vi "Ultrasonic Sensor simulationfirebase.(GroupDinithi).vi"() -> ()   [LabVIEW 2022 SP3]
uses:
  <vilib>/Analysis/2dsp.llb/Integral Method.ctl
  <vilib>/DAQmx/read.llb/DAQmx Read (Analog Wfm 1Chan NSamp).vi
  <vilib>/DAQmx/write.llb/DAQmx Write (Digital Bool 1Line 1Point).vi
  <vilib>/DAQmx/create/channels.llb/DAQmx Create Channel (DO-Digital Output).vi
  <vilib>/DAQmx/miscellaneous.llb/DAQmx Fill In Error Info.vi
  <vilib>/DAQmx/create/channels.llb/DAQmx Create Channel (AI-Voltage-Basic).vi
  <vilib>/DAQmx/configure/timing.llb/DAQmx Timing (Sample Clock).vi
  <vilib>/httpClient/PUTBuffer.vi
  <vilib>/Analysis/NI_AALPro.lvlib
  <vilib>/httpClient/LabVIEWHTTPClient.lvlib
panel:
  out "Numeric":dbl
  out "body":string
  in  "Cluster":T1
  out "Waveform Graph":waveform(dbl)(graph)
  in  "Number of Samples":dbl
  in  "sampling frequency":dbl
  in  "DAQmx Physical Channel 2":tag
  in  "DAQmx Physical Channel":tag
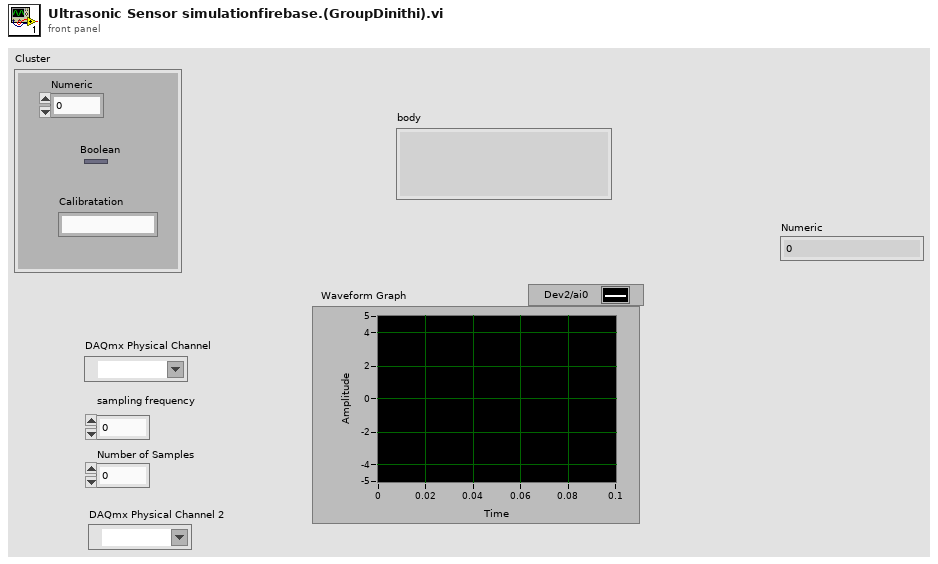
[diagram p1: front panel]
types:
  T1 = cluster{"Numeric":dbl, "Calibratation":string, "Boolean":bool}
  T2 = typedef "NI_AALPro.lvlib/Integral Method.ctl" = i32
  T3 = typedef "LabVIEWHTTPClient.lvlib/ClientHandle.ctl" = refnum<k1>
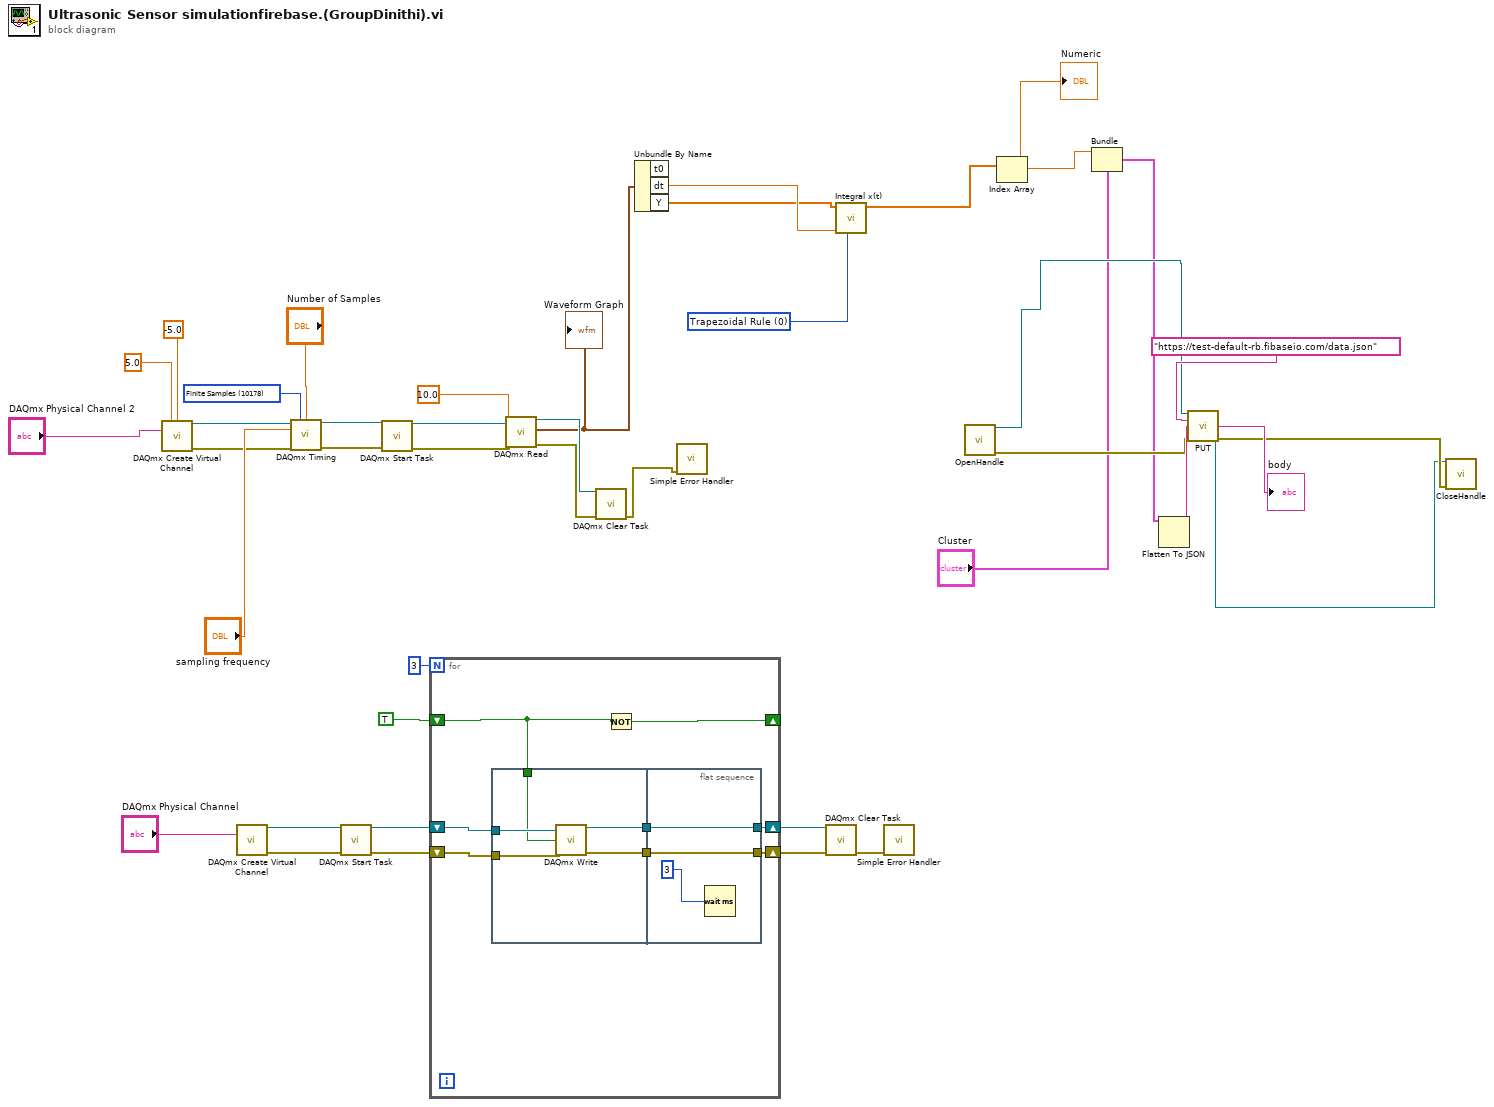
[diagram p0: block diagram]
diagram:
  w15 = T2 0 items=["Trapezoidal Rule", "Simpson's Rule", "Simpson's 3/8 Rule", "Bode Rule"] ("integration method")
  w28 = 10178 items=["Finite Samples"=10178, "Continuous Samples"=10123, "Hardware Timed Single Point"=12522] ("sample mode")
  n1 = call-poly <vilib>:"DAQmx Create Virtual Channel.vi"("maximum value"=5.0, "minimum value"=-5.0, "physical channels"="DAQmx Physical Channel 2") -> ("task out"=w27:refnum<k21>, "error out"=w26:errorcluster)  [unwired: 11 in]
  n2 = call-poly <vilib>:"DAQmx Create Virtual Channel.vi"("lines"="DAQmx Physical Channel") -> ("task out"=w40:refnum<k21>, "error out"=w41:errorcluster)  [unwired: 13 in]
  n3 = call-poly <vilib>:"DAQmx Timing.vi"("task/channels in"=w27, "sample mode"=w28, "samples per channel"="Number of Samples", "rate"="sampling frequency", "error in"=w26) -> ("task out"=w25:refnum<k21>, "error out"=w24:errorcluster)  [unwired: 9 in]
  n4 = call <vilib>:"DAQmx Start Task.vi"("task/channels in"=w40, "error in"=w41) -> ("task out"=w39:refnum<k21>, "error out"=w38:errorcluster)  [unwired: 12 in]
  n5 = call <vilib>:"DAQmx Start Task.vi"("task/channels in"=w25, "error in"=w24) -> ("task out"=w23:refnum<k21>, "error out"=w22:errorcluster)  [unwired: 12 in]
  n6 = for {
    N: 3 -> [_]
    shift-right: [w44] -> w35
    shift-left: w39 -> [w47]
    shift-right: [w45] -> w36
    shift-left: w38 -> [w46]
    shift-right: [w43] -> _
    shift-left: TRUE -> [w42]
    n7 = flat-sequence {
      tunnel: w47 -> [w54]
      tunnel: w46 -> [w53]
      tunnel: [w52] -> w49
      tunnel: [w51] -> w48
      tunnel: w42 -> [w50]
      tunnel: w49 -> [w56]
      tunnel: [w56] -> w45
      tunnel: w48 -> [w55]
      tunnel: [w55] -> w44
      frame #0 {
        n8 = call-poly <vilib>:"DAQmx Write.vi"("task/channels in"=w54, "data"=w50, "error in"=w53) -> ("task out"=w51:refnum<k21>, "error out"=w52:errorcluster)  [unwired: 10 in, 1 out]
      }
      frame #1 {
        n9 = Wait (ms)(milliseconds to wait=u32 3) -> ()  [unwired: 1 out]
      }
    }
    n10 = Not(x=w42) -> (.not. x?=w43:bool)
  }
  n11 = call-poly <vilib>:"DAQmx Read.vi"("task/channels in"=w23, "timeout"=10.0, "error in"=w22) -> ("task out"=w20:refnum<k21>, "data"=w12:waveform(dbl), "error out"=w19:errorcluster)  [unwired: 10 in]
  "Waveform Graph" <- w12
  n12 = call <vilib>:"DAQmx Clear Task.vi"("task in"=w20, "error in"=w19) -> ("error out"=w18:errorcluster)  [unwired: 13 in]
  n13 = Unbundle By Name(w12) -> ("dt"=w14:dbl, "Y"=w13:dbl[])  [unwired: 1 out]
  n14 = call <vilib>:"Simple Error Handler.vi"("error in (no error)"=w18) -> ()  [unwired: 4 in, 5 out]
  n15 = call <vilib>:"DAQmx Clear Task.vi"("task in"=w35, "error in"=w36) -> ("error out"=w34:errorcluster)  [unwired: 13 in]
  n16 = call <vilib>:"Integral x(t).vi"("integration method"=w15, "dt"=w14, "X"=w13) -> ("Integral X"=w11:dbl[])  [unwired: 7 in, 1 out]
  n17 = call <vilib>:"Simple Error Handler.vi"("error in (no error)"=w34) -> ()  [unwired: 4 in, 5 out]
  n18 = call <vilib>:"OpenHandle.vi"() -> ("client handle out"=w6:T3, "error out"=w7:errorcluster)  [unwired: 14 in]
  n19 = Index Array(array=w11) -> (element=w1:dbl)  [unwired: 1 in]
  "Numeric" <- w1
  n20 = Bundle(cluster="Cluster", "Numeric"=w1) -> (w2:T1)  [unwired: 2 in]
  n21 = Flatten To JSON(anything=w2) -> (JSON string=w8:string)  [unwired: 2 in, 1 out]
  n22 = call-poly <vilib>:"PUT.vi"("client handle"=w6, "url"="https://test-default-rb.fibaseio.com/data.json", "buffer"=w8, "error in (no error)"=w7) -> ("client handle out"=w4:T3, "body"=→"body":string, "error out"=w5:errorcluster)  [unwired: 8 in, 1 out]
  n23 = call <vilib>:"CloseHandle.vi"("client handle"=w4, "error in (no error)"=w5) -> ()  [unwired: 13 in, 1 out]
